vi "fg_interface.vi"(7 "fg_command":T3=enum."read", 8 "error in (no error)":errorcluster, 10 "interface [] in":T1[](array[typedef]), 11 "interface":T2) -> (0 "error out":errorcluster, 2 "interface [] out":T1[](array[typedef]), 3 "interface":T1)   [LabVIEW 2015, in "lv-interface-dom-nre.lvlib"]
uses:
  lv-interface-dom-nre.lvlib
  _controls/interface_refnum.ctl
  public/_controls/fg_command.ctl
  lv-interface-sub-common/_controls/interface_selection.ctl
  lv-interface-sub-common/lv-interface-sub-common.lvlib
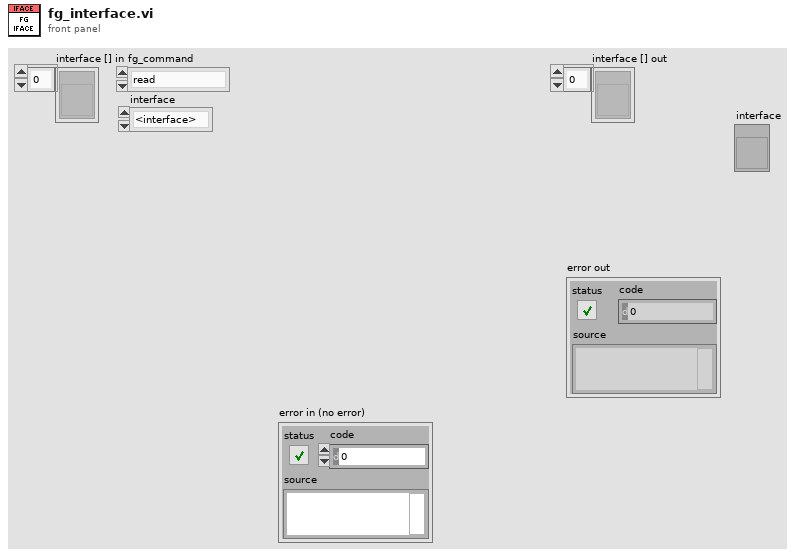
[diagram p1: front panel]
types:
  T1 = typedef "lv-interface-dom-nre.lvlib/interface_refnum.ctl" = refnum<vi>
  T2 = typedef "lv-interface-sub-common.lvlib/interface_selection.ctl" = enum16{"<interface>", "sub_interface_1", "sub_interface_2", "<null>"}
  T3 = typedef "lv-interface-dom-nre.lvlib/fg_command.ctl" = enum16{"<fg_command>", "initialize", "read", "write", "shutdown", "<null>"}
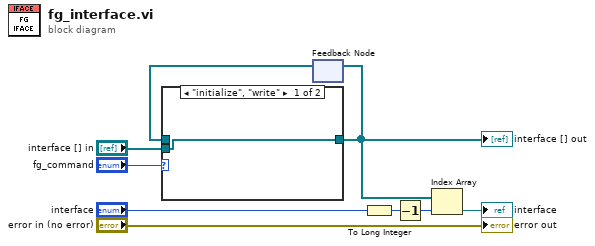
[diagram p0: block diagram]
diagram:
  n1 = feedback #1() -> (w7:T1[])  [unwired: 1 in]
  n2 = case shown="\"initialize\", \"write\"" "fg_command" {
    tunnel: "interface [] in" -> [w10 _]
    tunnel: [w10 w11] -> w6
    tunnel: w7 -> [_ w11]
    frame "initialize", "write" {
    }
    frame "read", Default {
    }
  }
  "interface [] out" <- w6
  n3 = feedback-in #1(w6) -> ()
  n4 = To Long Integer(number="interface") -> (32bit integer=w4:i32)
  n5 = Decrement(x=w4) -> (x-1=w2:i32)
  n6 = Index Array(array=w6, index=w2) -> (element=→"interface":T1)
  "error out" <- "error in (no error)"
